vi "KN-StringToAnnulusAndOptions.vi"(0 "String":string) -> (4 "ROI Descriptor":T6 {"Contours"."Type" items=["No Selection", "Point", "Line", "Rectangle", "Oval", "Polygon", "Freehand Region", "Annulus", "Unused2", "Unused3", "Broken Line", "Freehand Line", "Rotated Rectangle"]}, 6 "Option All":T5 {"Edge Options"."Edge Polarity" items=["All Edges", "Rising Edges", "Falling Edges"]; "Edge Options"."Minimum Edge Strength" format="%.2f"; "Edge Options"."Width" step=2; "Edge Options"."Kernel Size" step=2}, 8 "UI SHOW":T3 {"Edge Options"."Edge Polarity" items=["All Edges", "Rising Edges", "Falling Edges"]; "Edge Options"."Minimum Edge Strength" format="%.2f"; "Edge Options"."Width" step=2; "Edge Options"."Kernel Size" step=2}, 10 "Circle Fit Options":T4, 15 "Range (Threshold 1)":cluster{"Lower value":sgl, "Upper value":sgl}={"Lower value"=218.0, "Upper value"=255.0})   [LabVIEW 2015]
uses:
  <vilib>/vision/Measure.llb/Edge Options.ctl
  <vilib>/vision/Measure.llb/Edge Polarity.ctl
panel:
  out "已删除元素的数组子集":string[](array[string])
  out "已删除的部分":string[](array[string])
  out "All Data":string[](array[string])
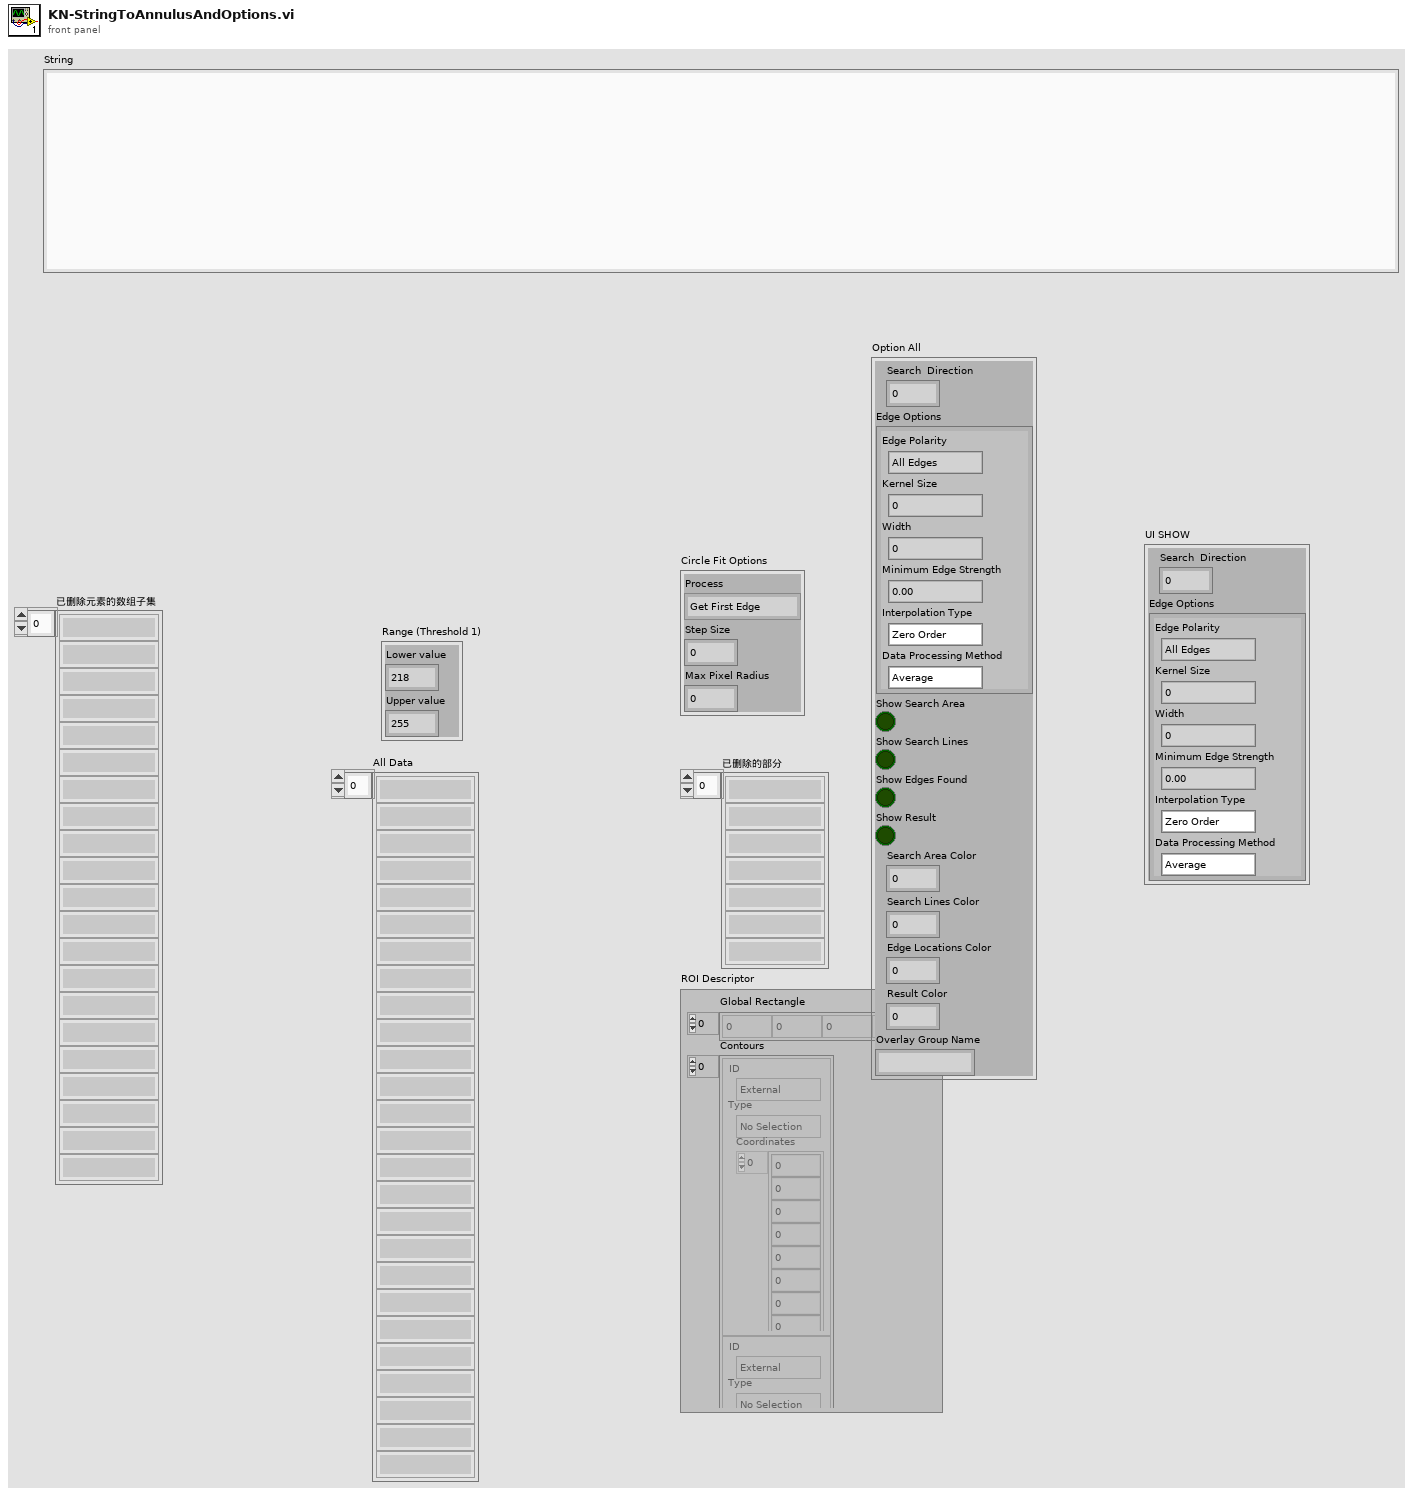
[diagram p1: front panel]
types:
  T1 = typedef "Edge Options.ctl" = cluster{"Edge Polarity":T2, "Kernel Size":u32, "Width":u32, "Minimum Edge Strength":sgl, "Interpolation Type":enum32{"Zero Order", "Bilinear", "Quadratic", "Cubic", "Bilinear Fixed"}, "Data Processing Method":enum32{"Average", "Median"}}
  T2 = typedef "Edge Polarity.ctl" = u32
  T3 = cluster{"Search  Direction":u32, "Edge Options":T1}
  T4 = cluster{"Process":enum16{"Get First Edge", "Get First + Last Edge", "Get All Edges", "Get Best Edge"}, "Step Size":i32, "Max Pixel Radius":i32}
  T5 = cluster{"Search  Direction":u32, "Edge Options":T1, "Show Search Area":bool, "Show Search Lines":bool, "Show Edges Found":bool, "Show Result":bool, "Search Area Color":u32, "Search Lines Color":u32, "Edge Locations Color":u32, "Result Color":u32, "Overlay Group Name":string}
  T6 = typedef "ROI Descriptor" = cluster{"Global Rectangle":i32[], "Contours":cluster{"ID":enum32{"External", "Internal"}, "Type":u32, "Coordinates":i32[]}[]}
  T7 = typedef "IMAQ Circle" = cluster{"Center X":i32, "Center Y":i32, "Inner Radius":i32, "Outer Radius":i32, "Start Angle":dbl, "End Angle":dbl}
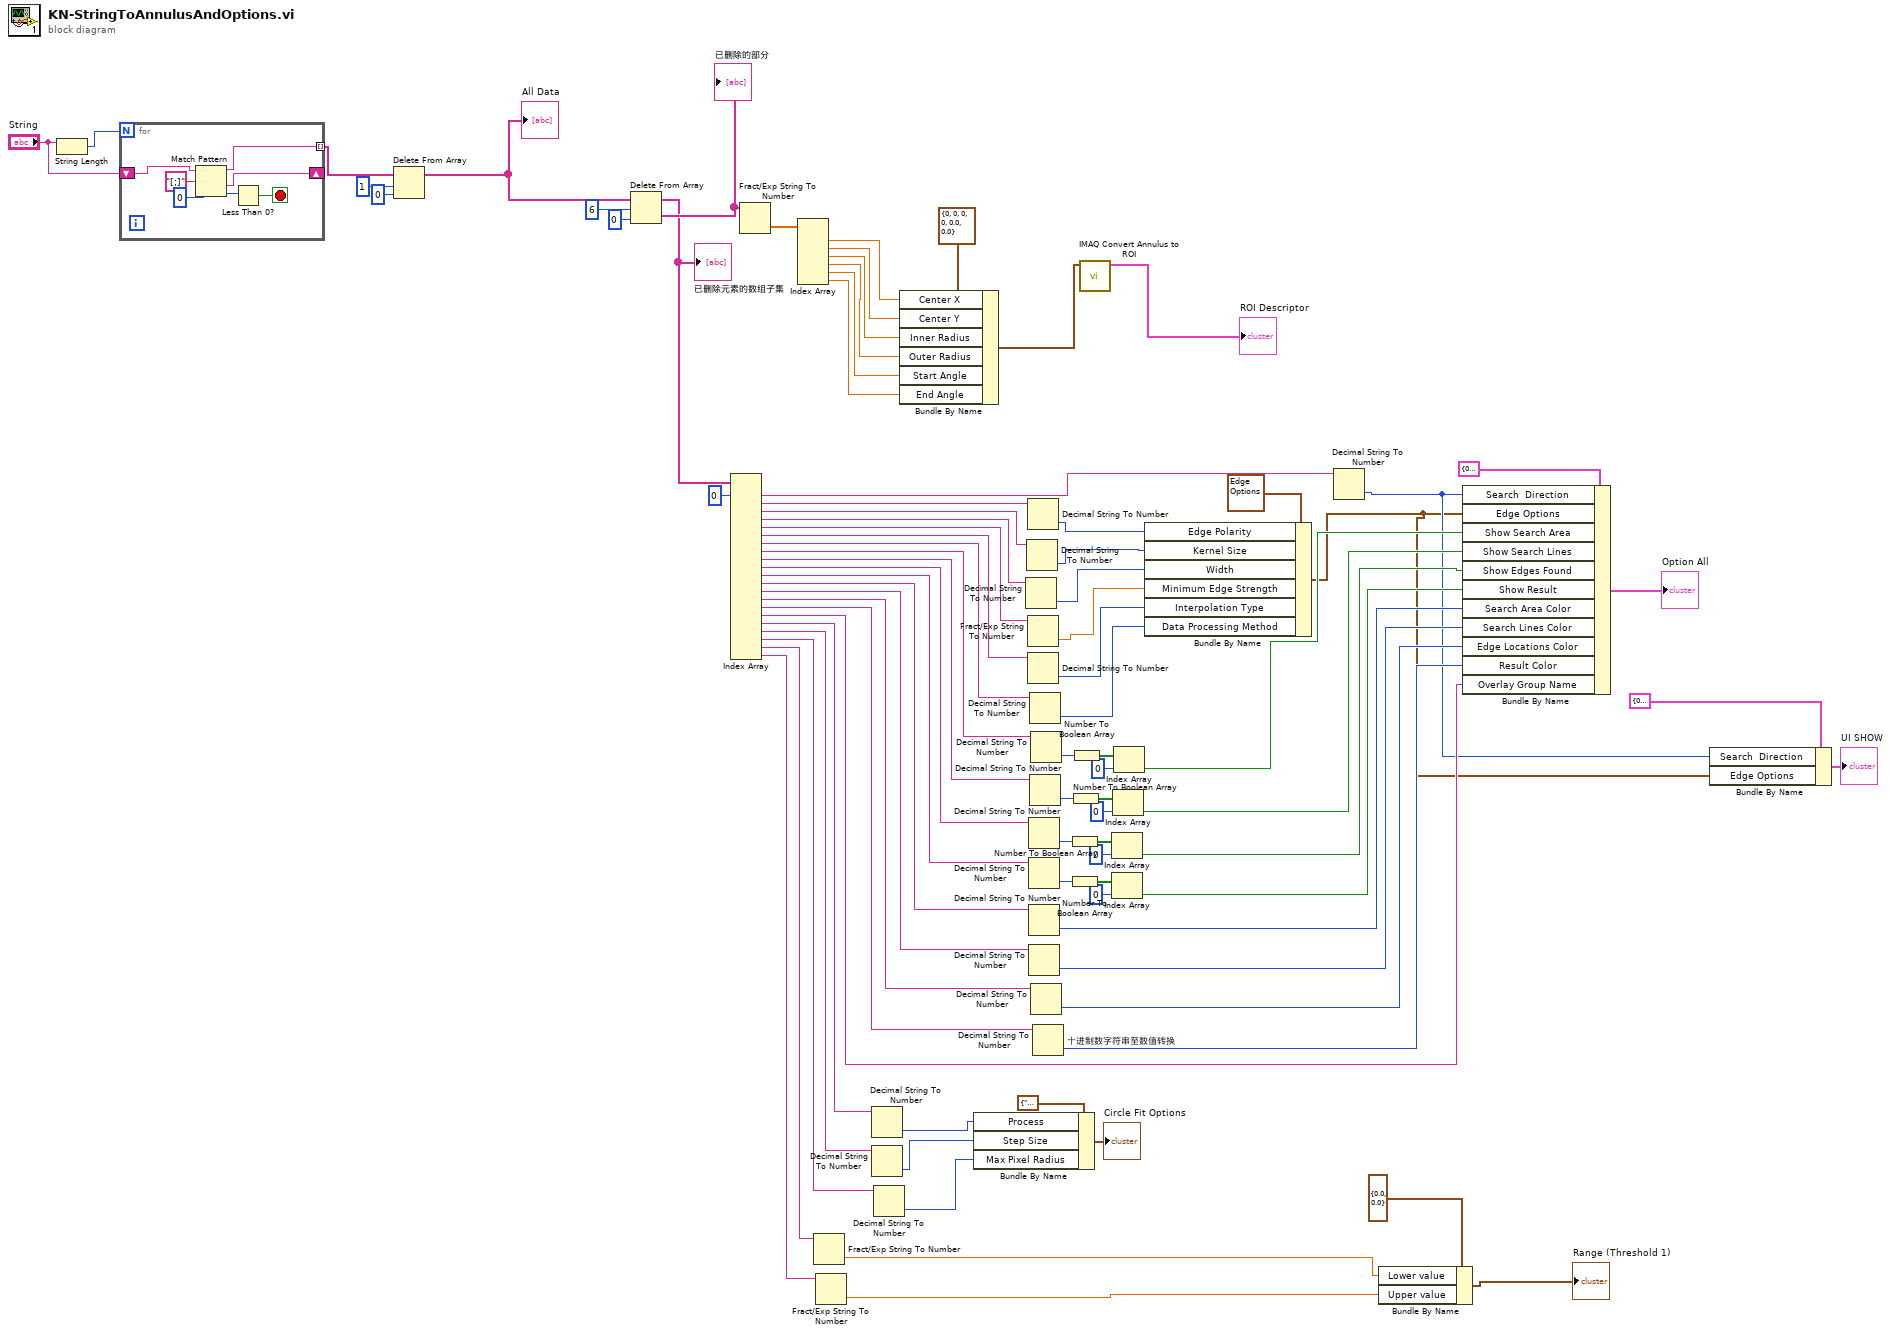
[diagram p0: block diagram]
diagram:
  n1 = String Length(string="String") -> (length=w83:i32)
  n2 = for {
    N: w83 -> [_]
    shift-right: [w86] -> _
    shift-left: "String" -> [w87]
    tunnel: [w85] -> w82 mode=indexing
    stop <- w88 stop-if-true
    n3 = Match Pattern(string=w87, regular expression="[;]" ("正则表达式"), offset (0)=0 ("偏移量(0)")) -> (before substring=w85:string, after substring=w86:string, offset past match=w89:i32)  [unwired: 1 out]
    n4 = Less Than 0?(x=w89) -> (x < 0?=w88:bool)
  }
  n5 = Delete From Array(array=w82, length=1 ("长度"), index=0 ("索引")) -> (array with subset deleted=w79:string[])  [unwired: 1 out]
  "All Data" <- w79
  n6 = Delete From Array(array=w79, length=6 ("长度"), index=0 ("索引")) -> (deleted portion=w76:string[], array with subset deleted=w69:string[])
  "已删除的部分" <- w76
  "已删除元素的数组子集" <- w69
  n7 = Index Array(array=w69, index #1=0 ("索引")) -> (element #1=w65:string, element #2=w64:string, element #3=w62:string, element #4=w60:string, element #5=w58:string, element #6=w56:string, element #7=w55:string, element #8=w52:string, element #9=w39:string, element #10=w38:string, element #11=w37:string, element #12=w33:string, element #13=w32:string, element #14=w31:string, element #15=w30:string, element #16=w25:string, element #17=w13:string, element #18=w11:string, element #19=w10:string, element #20=w6:string, element #21=w5:string)  [unwired: 20 in]
  n8 = Fract/Exp String To Number(string=w76) -> (number=w75:dbl[])  [unwired: 3 in, 1 out]
  n9 = Index Array(array=w75) -> (element #1=w22:dbl, element #2=w21:dbl, element #3=w23:dbl, element #4=w20:dbl, element #5=w73:dbl, element #6=w72:dbl)  [unwired: 6 in]
  n10 = Fract/Exp String To Number(string=w6) -> (number=w17:dbl)  [unwired: 3 in, 1 out]
  n11 = Fract/Exp String To Number(string=w5) -> (number=w16:dbl)  [unwired: 3 in, 1 out]
  n12 = Decimal String To Number ("十进制数字符串至数值转换")(string=w13) -> (number=w12:i32)  [unwired: 2 in, 1 out]
  n13 = Decimal String To Number ("十进制数字符串至数值转换")(string=w11) -> (number=w9:i32)  [unwired: 2 in, 1 out]
  n14 = Decimal String To Number ("十进制数字符串至数值转换")(string=w10) -> (number=w8:i32)  [unwired: 2 in, 1 out]
  n15 = Bundle By Name(cluster=T7 {"Center X"=0, "Center Y"=0, "Inner Radius"=0, "Outer Radius"=0, "Start Angle"=0.0, "End Angle"=0.0} ("Annulus"), "Center X"=w22, "Center Y"=w21, "Inner Radius"=w23, "Outer Radius"=w20, "Start Angle"=w73, "End Angle"=w72) -> (w71:T7)
  n16 = Bundle By Name(cluster=T4 {"Process"=enum."Get First Edge", "Step Size"=10, "Max Pixel Radius"=3} ("Circle Fit Options"), "Process"=w12, "Step Size"=w9, "Max Pixel Radius"=w8) -> (→"Circle Fit Options":T4)
  n17 = Decimal String To Number(string=w60) -> (number=w59:i32)  [unwired: 2 in, 1 out]
  n18 = Decimal String To Number(string=w62) -> (number=w61:i32)  [unwired: 2 in, 1 out]
  n19 = Decimal String To Number(string=w64) -> (number=w63:i32)  [unwired: 2 in, 1 out]
  n20 = Fract/Exp String To Number(string=w58) -> (number=w57:dbl)  [unwired: 3 in, 1 out]
  n21 = Decimal String To Number(string=w56) -> (number=w54:i32)  [unwired: 2 in, 1 out]
  n22 = Decimal String To Number(string=w38) -> (number=w45:i32)  [unwired: 2 in, 1 out]
  n23 = Decimal String To Number(string=w37) -> (number=w40:i32)  [unwired: 2 in, 1 out]
  n24 = Decimal String To Number(string=w33) -> (number=w29:i32)  [unwired: 2 in, 1 out]
  n25 = Decimal String To Number(string=w32) -> (number=w28:i32)  [unwired: 2 in, 1 out]
  n26 = Decimal String To Number(string=w55) -> (number=w53:i32)  [unwired: 2 in, 1 out]
  n27 = Decimal String To Number(string=w39) -> (number=w46:i32)  [unwired: 2 in, 1 out]
  n28 = Decimal String To Number(string=w52) -> (number=w51:i32)  [unwired: 2 in, 1 out]
  n29 = Decimal String To Number(string=w31) -> (number=w27:i32)  [unwired: 2 in, 1 out]
  n30 = Decimal String To Number "十进制数字符串至数值转换"(string=w30) -> (number=w26:i32)  [unwired: 2 in, 1 out]
  n31 = Number To Boolean Array(number=w45) -> (Boolean array=w44:bool[])
  n32 = Number To Boolean Array(number=w40) -> (Boolean array=w41:bool[])
  n33 = Number To Boolean Array(number=w46) -> (Boolean array=w47:bool[])
  n34 = Number To Boolean Array(number=w51) -> (Boolean array=w50:bool[])
  n35 = call "IMAQ Convert Annulus to ROI"("Annulus"=w71) -> ("ROI Descriptor"=→"ROI Descriptor":T6)  [unwired: 8 in, 1 out]
  n36 = Index Array(array=w44, index=0 ("索引")) -> (element=w35:bool)
  n37 = Index Array(array=w41, index=0 ("索引")) -> (element=w34:bool)
  n38 = Index Array(array=w47, index=0 ("索引")) -> (element=w36:bool)
  n39 = Index Array(array=w50, index=0 ("索引")) -> (element=w19:bool)
  n40 = Bundle By Name(cluster=T1 {"Edge Polarity"=0, "Kernel Size"=0, "Width"=0, "Minimum Edge Strength"=0.0, "Interpolation Type"=enum."Bilinear Fixed", "Data Processing Method"=enum."Average"} ("Edge Options"), "Edge Polarity"=w63, "Kernel Size"=w61, "Width"=w59, "Minimum Edge Strength"=w57, "Interpolation Type"=w54, "Data Processing Method"=w53) -> (w2:T1)
  n41 = Decimal String To Number(string=w65) -> (number=w3:i32)  [unwired: 2 in, 1 out]
  n42 = Bundle By Name(cluster=cluster{"Lower value":sgl, "Upper value":sgl} {"Lower value"=0.0, "Upper value"=0.0} ("Red or Hue Range (Color Threshold 1)"), "Lower value"=w17, "Upper value"=w16) -> (→"Range (Threshold 1)":cluster{"Lower value":sgl, "Upper value":sgl})
  n43 = Bundle By Name(cluster=T5 {"Search  Direction"=0, "Edge Options"={"Edge Polarity"=0, "Kernel Size"=0, "Width"=0, "Minimum Edge Strength"=0.0, "Interpolation Type"=enum."Bilinear Fixed", "Data Processing Method"=enum."Average"}, "Show Search Area"=FALSE, "Show Search Lines"=FALSE, "Show Edges Found"=FALSE, "Show Result"=TRUE, "Search Area Color"=65280, "Search Lines Color"=255, "Edge Locations Color"=16776960, "Result Color"=16711680, "Overlay Group Name"=""} ("Options (Find Circular Edge 1)"), "Search  Direction"=w3, "Edge Options"=w2, "Show Search Area"=w19, "Show Search Lines"=w36, "Show Edges Found"=w35, "Show Result"=w34, "Search Area Color"=w29, "Search Lines Color"=w28, "Edge Locations Color"=w27, "Result Color"=w26, "Overlay Group Name"=w25) -> (→"Option All":T5)
  n44 = Bundle By Name(cluster=T3 {"Search  Direction"=0, "Edge Options"={"Edge Polarity"=0, "Kernel Size"=0, "Width"=0, "Minimum Edge Strength"=0.0, "Interpolation Type"=enum."Bilinear Fixed", "Data Processing Method"=enum."Average"}} ("Options (Find Circular Edge 1)"), "Search  Direction"=w3, "Edge Options"=w2) -> (→"UI SHOW":T3)
